vi "New.vi"(8 "error in (no error)":errorcluster) -> (0 "error out":errorcluster, 3 "Beam out":refnum<class "Beam.lvclass">)   [LabVIEW 2019, in "Beam.lvclass"]
uses:
  Beam.lvclass
  Beam.lvclass/Beam.ctl
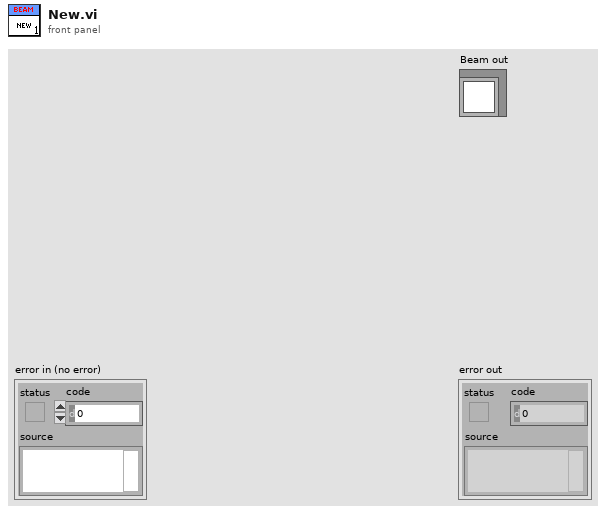
[diagram p1: front panel]
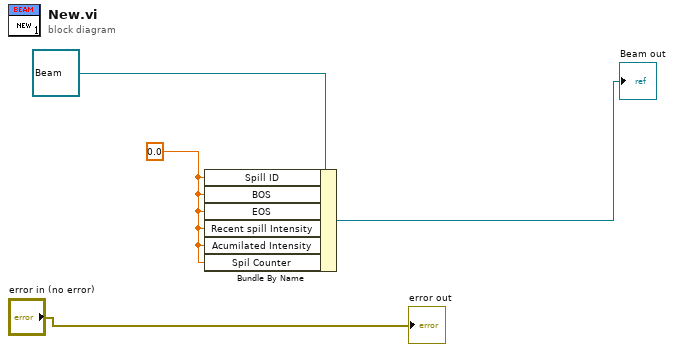
[diagram p0: block diagram]
diagram:
  w2 = 0.0 ("Spill ID")
  n1 = Bundle By Name(cluster=refnum<class "Beam.lvclass"> refnum ("Beam.lvclass"), "Spill ID"=w2, "BOS"=w2, "EOS"=w2, "Recent spill Intensity"=w2, "Acumilated Intensity"=w2, "Spil Counter"=w2) -> (→"Beam out":refnum<class "Beam.lvclass">)
  "error out" <- "error in (no error)"
